vi "Substitute Actor.vi"(10 "Substitute Actor in":refnum<class "Actor.lvclass">, 11 "Current Connect Command":refnum<class "Connect Command.lvclass">) -> (0 "error out":errorcluster, 2 "Substitute Actor out":refnum<class "Actor.lvclass">)   [LabVIEW 2013]
doc: "(<B>Filename</B>: Actor Framework.lvlib:Actor.lvclass:Substitute Actor.vi)\n\nThis method copies information from the <b>Current Actor</b> to the <b>Substitute Actor</b>, including the to-self and the to-caller queue references. The purpose of this function is to allow an actor to define a method that replaces itself with another actor, useful for implementing a State Pattern Actor. Child classes should override this method to copy any additional fields that they need from the current to the substitute.\n\nThis method may return error code 678010: Illegal substitution. Overrides of this method may choose to return this error if the new actor is not one that is an appropriate substitute for the current actor, for whatever standards of \"appropriate\" are chosen for the current actor. If returning an error, override VIs should return the unmodified <b>Current Actor</b> as <b>Substitute Actor out</b>."
uses:
  <vilib>/ActorFramework/Actor/Actor.lvclass
  Connect Command.lvclass
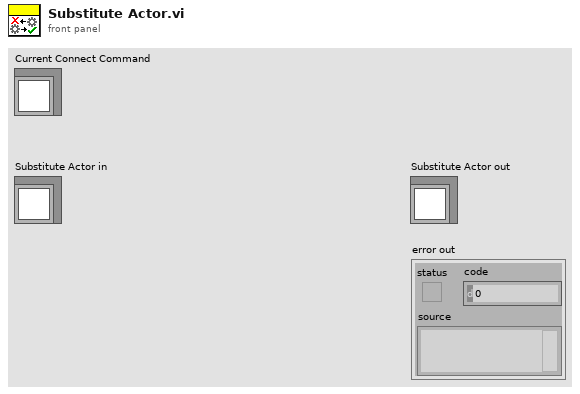
[diagram p1: front panel]
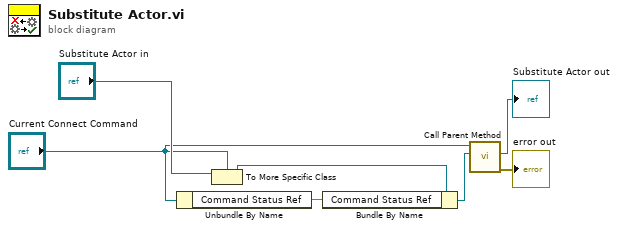
[diagram p0: block diagram]
diagram:
  n1 = Unbundle By Name("Current Connect Command") -> ("Command Status Ref"=w1)
  n2 = To More Specific Class(target class="Current Connect Command", reference="Substitute Actor in") -> (specific class reference=w5:refnum<class "Connect Command.lvclass">)  [unwired: 1 in, 1 out]
  n3 = Bundle By Name(cluster=w5, "Command Status Ref"=w1) -> (w2:refnum<class "Connect Command.lvclass">)
  n4 = call-parent "Call Parent Method"("Substitute Actor in"=w2, "Current Actor"="Current Connect Command") -> ("error out"=→"error out":errorcluster, "Substitute Actor out"=→"Substitute Actor out":refnum<class "Actor.lvclass">)  [unwired: 8 in]
